vi "FilieIO.vi"() -> ()   [LabVIEW 2012]
uses:
  <vilib>/Utility/file.llb/Read From Spreadsheet File (string).vi
  <vilib>/Utility/file.llb/Write To Spreadsheet File (string).vi
panel:
  in  "subarray":string[](array[string])
  in  "String":string="B01-0995-05"
  out "all rows":string[][](array[string])
  in  "OK Button":bool
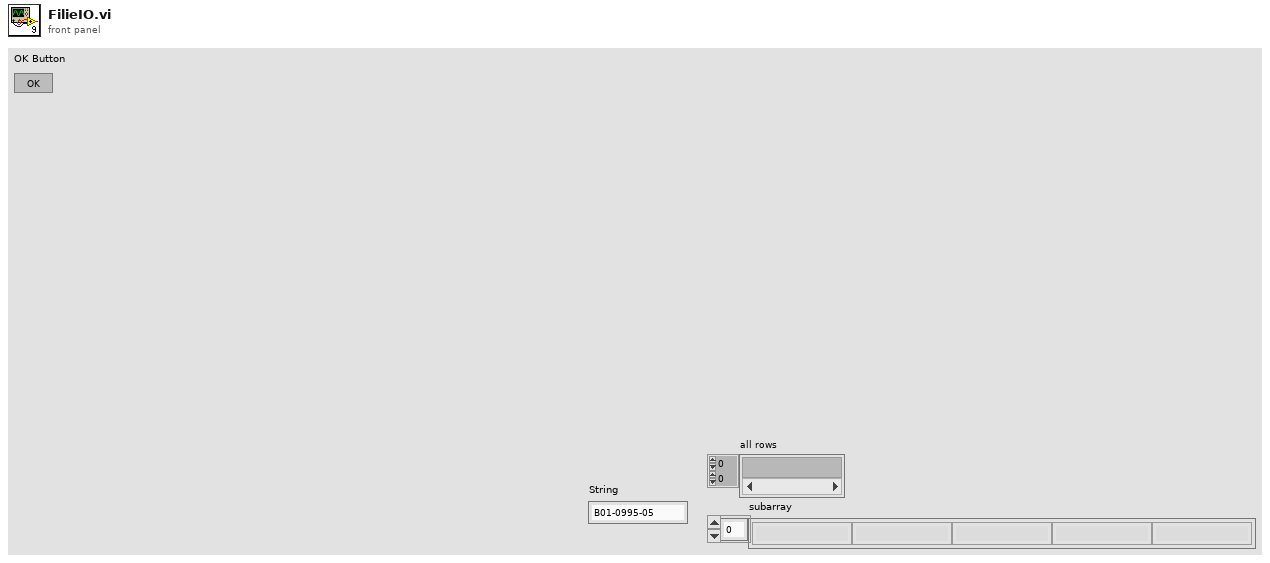
[diagram p1: front panel]
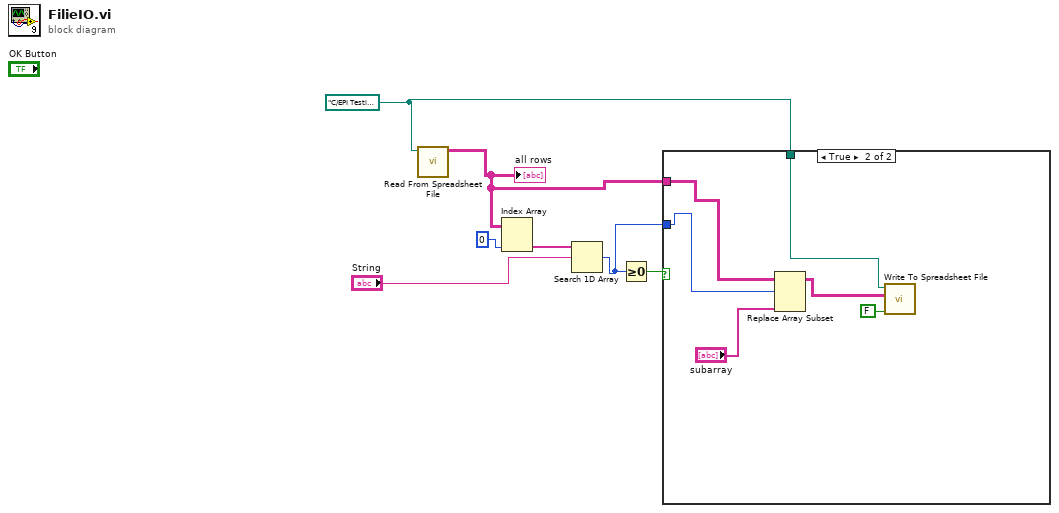
[diagram p0: block diagram]
diagram:
  w3 = path "C:/EPI Testing/Wafer Data.txt" ("file path (dialog if empty)")
  n1 = call-poly <vilib>:"Read From Spreadsheet File.vi"("file path (dialog if empty)"=w3) -> ("all rows"=w4:string[][])  [unwired: 6 in, 4 out]
  "all rows" <- w4
  n2 = Index Array(array=w4, index (col)=0 ("index (row)")) -> (element=w7:string[])  [unwired: 1 in]
  n3 = Search 1D Array(1D array=w7, element="String") -> (index of element=w2:i32)  [unwired: 1 in]
  n4 = Greater Or Equal To 0?(x=w2) -> (x >= 0?=w1:bool)
  n5 = case shown="True" w1 {
    tunnel: w4 -> [_ w13]
    tunnel: w2 -> [_ w12]
    tunnel: w3 -> [_ w8]
    frame False {
    }
    frame True {
      n6 = Replace Array Subset(array=w13, new element="subarray", index (row)=w12) -> (w10:string[][])  [unwired: 1 in]
      n7 = call-poly <vilib>:"Write To Spreadsheet File.vi"("append to file? (new file:F)"=FALSE, "2D data"=w10, "file path (dialog if empty)"=w8) -> ()  [unwired: 5 in, 1 out]
    }
  }
